vi "Initialization VI.vi"(8 "error in (no error)":errorcluster, 10 "Custom XML":string, 11 "Device Item Ref in":T1 format="%.0x") -> (0 "error out":errorcluster, 3 "Device Item Ref out":T1 format="%.0x")   [LabVIEW 2020, in "Waveform Analog Output System Explorer.lvlib"]
uses:
  Waveform Analog Output System Explorer.lvlib
  <vilib>/NI VeriStand/Custom Device API/Custom Device Item Ref.ctl
  <vilib>/NI VeriStand/Custom Device API/Custom Device Channel.ctl
  <vilib>/NI VeriStand/Custom Device API/Custom Device Channel Type.ctl
  Number of AO Channels.ctl
  Shared/Constants.vi
  <vilib>/NI VeriStand/Custom Device API/Set Item Property (Variant).vi
  <vilib>/NI VeriStand/Custom Device API/Set Item Property (U16).vi
  <vilib>/NI VeriStand/Custom Device API/Custom Device API.lvlib
  Shared/Waveform Analog Output Shared.lvlib
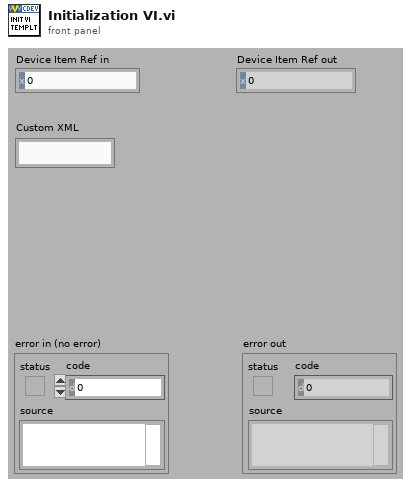
[diagram p1: front panel]
types:
  T1 = typedef "Custom Device API.lvlib/Custom Device Item Ref.ctl" = u64
  T2 = typedef "Custom Device API.lvlib/Custom Device Channel.ctl" = cluster{"Type":T3, "Units":string, "Default Value":dbl, "Faultable":bool, "Scalable":bool}
  T3 = typedef "Custom Device API.lvlib/Custom Device Channel Type.ctl" = enum16{"Input", "Output"}
  T4 = typedef "Waveform Analog Output System Explorer.lvlib/Number of AO Channels.ctl" = u16
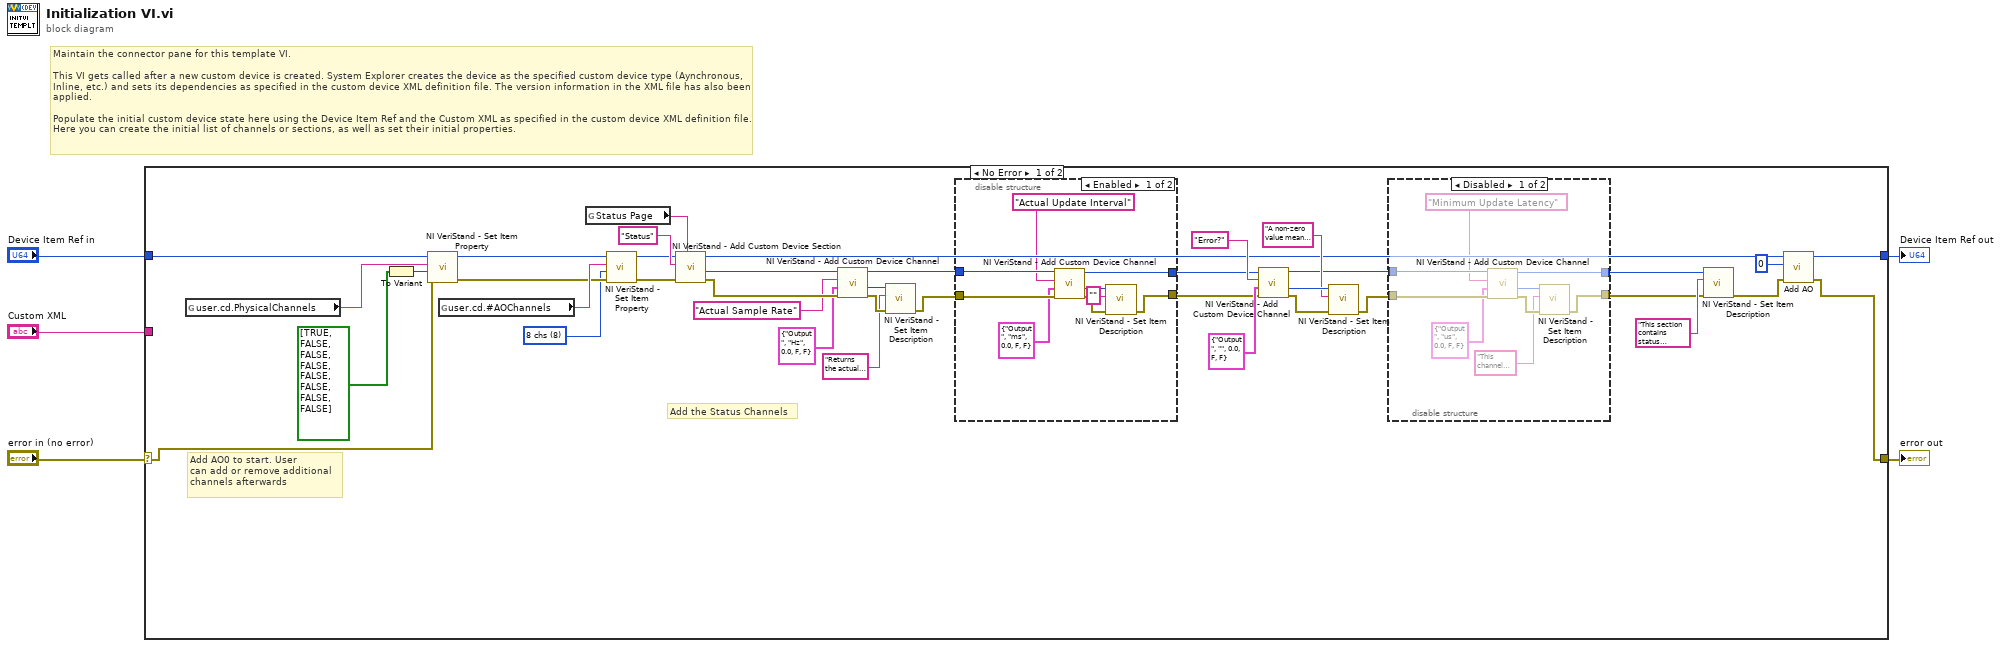
[diagram p0: block diagram]
diagram:
  # "Maintain the connector pane for this template VI.\n\nThis VI gets called after a new custom device is created. System Explorer creates the device as the specified custom device type (Aynchronous, Inline, etc.) and sets its dependencies as specified in the custom device XML definition file. The version information in the XML file has also been applied.\n\nPopulate the initial custom device state here using the Device Item Ref and the Custom XML as specified in the custom device XML definition file. Here you can create the initial list of channels or sections, as well as set their initial properties."
  n1 = case shown="No Error" "error in (no error)" {
    selector: "error in (no error)" -> [w43 w68]
    tunnel: [w11 w68] -> w5
    tunnel: [w12 w67] -> w3
    tunnel: "Device Item Ref in" -> [w44 w67]
    tunnel: "Custom XML" -> [_ _]
    frame No Error {
      w15 = T4 8 items=["2 chs"=2, "4 chs"=4, "8 chs"=8, "32 chs"=32, "64 chs"=64] ("Number of AO Channels")
      # "Add the Status Channels"
      # "Add AO0 to start. User\ncan add or remove additional\nchannels afterwards"
      n2 = global read "Constants.vi" "user.cd.PhysicalChannels"() -> (w37:string)
      n3 = To Variant(anything=bool[] [TRUE, FALSE, FALSE, FALSE, FALSE, FALSE, FALSE, FALSE]) -> (Variant=w36:variant)
      n4 = call-poly <vilib>:"NI VeriStand - Set Item Property.vi"("error in (no error)"=w43, "Value"=w36, "Property Name"=w37, "Item Ref in"=w44) -> ("error out"=w17:errorcluster, "Item Ref out"=w19:T1)  [unwired: 5 in, 1 out]
      n5 = global read "Constants.vi" "user.cd.#AOChannels"() -> (w20:string)
      n6 = global read "Constants.vi" "Status Page"() -> (w25:string)
      n7 = call-poly <vilib>:"NI VeriStand - Set Item Property.vi"("error in (no error)"=w17, "Value"=w15, "Property Name"=w20, "Item Ref in"=w19) -> ("error out"=w16:errorcluster, "Item Ref out"=w18:T1)  [unwired: 5 in, 1 out]
      n8 = call <vilib>:"NI VeriStand - Add Custom Device Section.vi"("GUID (Default Section)"=w25, "error in (no error)"=w16, "Section Name"="Status", "Parent Ref in"=w18) -> ("error out"=w40:errorcluster, "Section Ptr"=w41:T1, "Parent Ref out"=w13:T1)  [unwired: 4 in, 1 out]
      n9 = call <vilib>:"NI VeriStand - Add Custom Device Channel.vi"("error in (no error)"=w40, "Channel"=T2 {"Type"=enum."Output", "Units"="Hz", "Default Value"=0.0, "Faultable"=FALSE, "Scalable"=FALSE}, "Channel Name"="Actual Sample Rate", "Parent Ref in"=w41) -> ("error out"=w28:errorcluster, "Channel Ref"=w29:T1, "Parent Ref out"=w8:T1)  [unwired: 4 in, 1 out]
      n10 = call <vilib>:"NI VeriStand - Set Item Description.vi"("error in (no error)"=w28, "Description"="Returns the actual sample rate that the DAQ card is using to generate the waveforms. This value is returned during initialization and will not change as the system runs.", "Item Ref in"=w29) -> ("error out"=w9:errorcluster)  [unwired: 6 in, 2 out]
      n11 = disable-structure shown="Enabled" {
        disable-tunnel: w8 -> [w53 w55]
        disable-tunnel: w9 -> [w52 w54]
        disable-tunnel: [w47 w55] -> w7
        disable-tunnel: [w46 w54] -> w6
        frame Enabled {
          n12 = call <vilib>:"NI VeriStand - Add Custom Device Channel.vi"("error in (no error)"=w52, "Channel"=T2 {"Type"=enum."Output", "Units"="ms", "Default Value"=0.0, "Faultable"=FALSE, "Scalable"=FALSE}, "Channel Name"="Actual Update Interval", "Parent Ref in"=w53) -> ("error out"=w48:errorcluster, "Channel Ref"=w49:T1, "Parent Ref out"=w47:T1)  [unwired: 4 in, 1 out]
          n13 = call <vilib>:"NI VeriStand - Set Item Description.vi"("error in (no error)"=w48, "Description"="", "Item Ref in"=w49) -> ("error out"=w46:errorcluster)  [unwired: 6 in, 2 out]
        }
        frame Disabled {
        }
      }
      n14 = call <vilib>:"NI VeriStand - Add Custom Device Channel.vi"("error in (no error)"=w6, "Channel"=T2 {"Type"=enum."Output", "Units"="", "Default Value"=0.0, "Faultable"=FALSE, "Scalable"=FALSE}, "Channel Name"="Error?", "Parent Ref in"=w7) -> ("error out"=w31:errorcluster, "Channel Ref"=w32:T1, "Parent Ref out"=w24:T1)  [unwired: 4 in, 1 out]
      n15 = call <vilib>:"NI VeriStand - Set Item Description.vi"("error in (no error)"=w31, "Description"="A non-zero value means an error has occurred and the custom device has shut down", "Item Ref in"=w32) -> ("error out"=w23:errorcluster)  [unwired: 6 in, 2 out]
      n16 = disable-structure shown="Disabled" {
        disable-tunnel: w24 -> [w64 w66]
        disable-tunnel: w23 -> [w63 w65]
        disable-tunnel: [w57 w66] -> w22
        disable-tunnel: [w56 w65] -> w21
        frame Disabled {
          n17 = call <vilib>:"NI VeriStand - Add Custom Device Channel.vi"("error in (no error)"=w63, "Channel"=T2 {"Type"=enum."Output", "Units"="us", "Default Value"=0.0, "Faultable"=FALSE, "Scalable"=FALSE}, "Channel Name"="Minimum Update Latency", "Parent Ref in"=w64) -> ("error out"=w59:errorcluster, "Channel Ref"=w60:T1, "Parent Ref out"=w57:T1)  [unwired: 4 in, 1 out]
          n18 = call <vilib>:"NI VeriStand - Set Item Description.vi"("error in (no error)"=w59, "Description"="This channel outputs the minimum latency expected for new parameter values to update the waveform. This latency is calculated based on the current write location in the output buffer when a parameter value change occurs. Note that the latency can be slightly higher based on write location of the HW buffer.", "Item Ref in"=w60) -> ("error out"=w56:errorcluster)  [unwired: 6 in, 2 out]
        }
        frame Enabled {
        }
      }
      n19 = call <vilib>:"NI VeriStand - Set Item Description.vi"("error in (no error)"=w21, "Description"="This section contains status channels useful for tracking the health of this custom device.", "Item Ref in"=w22) -> ("error out"=w10:errorcluster)  [unwired: 6 in, 2 out]
      n20 = call "Add AO.vi"("error in (no error)"=w10, "Physical Channel Number"=0, "Device Item Ref in"=w13) -> ("error out"=w11:errorcluster, "Parent Ref out"=w12:T1)  [unwired: 7 in]
    }
    frame Error {
    }
  }
  "error out" <- w5
  "Device Item Ref out" <- w3
